vi "Digital Telemetry.vi"() -> ()   [LabVIEW 2020]
uses:
  <vilib>/MakerHub/LINX/Private/Type Defs/Peripheral.ctl
  <vilib>/MakerHub/LINX/Public/Peripherals/Digital/Digital Read 1 Chan.vi
  <vilib>/MakerHub/LINX/Public/Peripherals/Digital/Digital Write 1 Chan.vi
  <vilib>/MakerHub/LINX/Public/Peripherals/Digital/Digital Read N Chans.vi
  <vilib>/MakerHub/LINX/Public/Peripherals/Digital/Digital Write N Chans.vi
  <vilib>/MakerHub/LINX/Private/Local IO/LinxDigitalRead.vi
  <vilib>/MakerHub/LINX/Private/Local IO/LinxDigitalWrite.vi
  <vilib>/MakerHub/LINX/Public/Utilities/Open Local.vi
  <vilib>/MakerHub/LINX/Private/Utilties/Generate Error.vi
  <vilib>/MakerHub/LINX/LMH-LINX.lvlib
panel:
  out "Error Out 3":errorcluster
  out "Numeric":i32
  in  "DO Channel":u8
  out "Error Out":errorcluster
  in  "Write Value?":bool
  in  "Write All?":bool
  in  "Output Value":bool
  out "Numeric 2":u8
  out "Error Out 2":errorcluster
  out "Values":bool[](array[boolean])
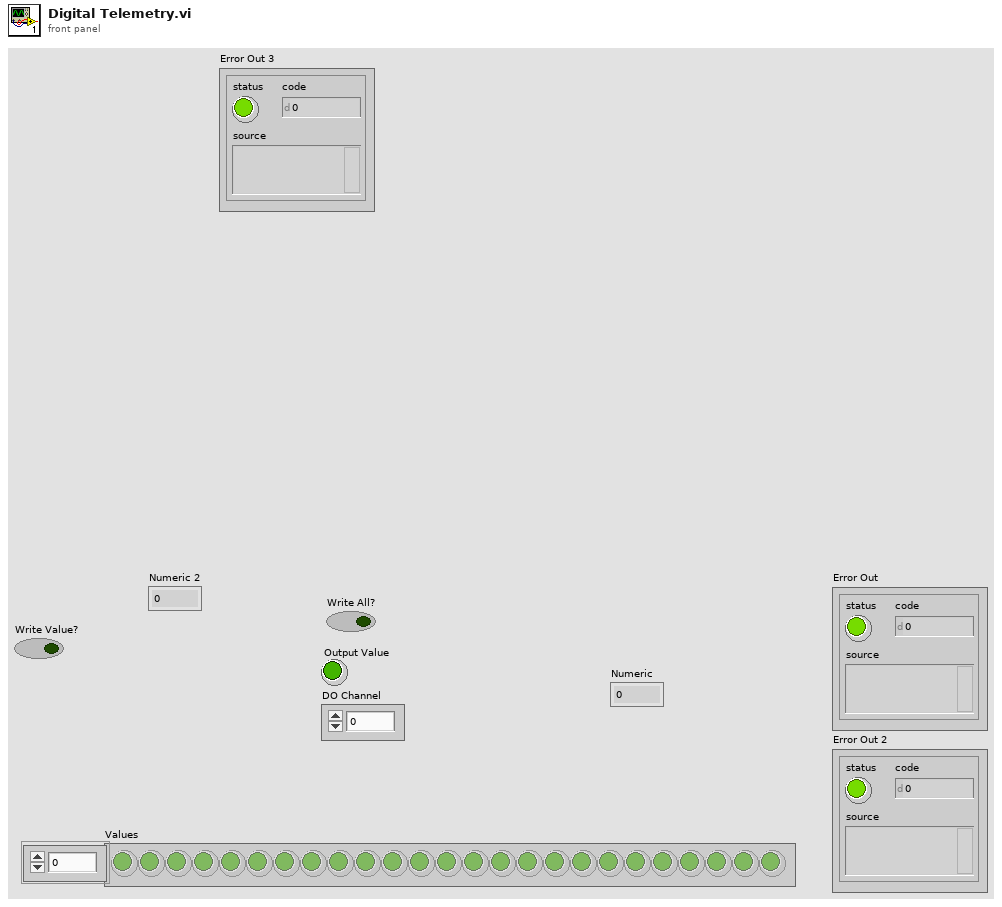
[diagram p1: front panel]
types:
  T1 = typedef "LMH-LINX.lvlib/LINX Ref.ctl" = cluster{"IO":T2, "Interface":T3, "LINX Device Config":T4}
  T2 = typedef "LMH-LINX.lvlib/Platform.ctl" = enum16{"Remote", "Local"}
  T3 = typedef "LMH-LINX.lvlib/Interface.ctl" = enum16{"Serial", "TCP"}
  T4 = typedef "LMH-LINX.lvlib/Device.lvlib/LINX Device Config.ctl" = cluster{"Interface":T3, "COM Port":refnum<visa-resource-name>, "TCP Configuration":T5, "Device Family":u8, "Device ID":u8, "Device Name":string, "TCP Ref":refnum<k5>, "Channels":T6}
  T5 = typedef "LMH-LINX.lvlib/Device.lvlib/TCP Config.ctl" = cluster{"IP Address":string, "Port":u16}
  T6 = typedef "LMH-LINX.lvlib/Channels.ctl" = cluster{"DI":u8[], "DO":u8[], "AI":u8[], "AO":u8[], "PWM":u8[], "QE":u8[], "UART":u8[], "I2C 2":u8[], "SPI":u8[], "CAN":u8[], "Servo":u8[], "AI Ref (V)":dbl, "AI Resolution (Bits)":u8, "AO Ref (V)":dbl, "AO Resolution (Bits)":u8}
  T7 = typedef "LMH-LINX.lvlib/Peripheral.ctl" = enum8{"DI", "DO", "AI", "AO", "PWM", "QE", "UART", "I2C", "SPI", "CAN", "Servo"}
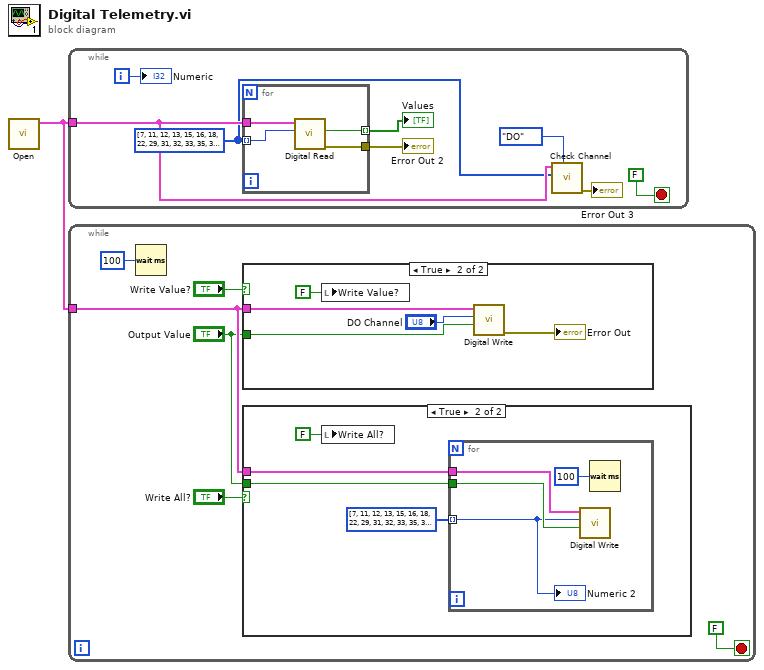
[diagram p0: block diagram]
diagram:
  n1 = call-poly <vilib>:"Open.vi"() -> ("LINX Resource"=w1:T1)  [unwired: 9 in, 2 out]
  n2 = while {
    tunnel: w1 -> [w4]
    i -> [w6]
    stop <- FALSE stop-if-true
    w2 = u8[] [7, 11, 12, 13, 15, 16, 18, 22, 29, 31, 32, 33, 35, 36, 37, 38, 40] ("DI Channels")
    n3 = for {
      tunnel: [w13] -> w9 mode=indexing
      tunnel: [w12] -> w8
      tunnel: w2 -> [w11] mode=indexing
      tunnel: w4 -> [w10]
      n4 = call-poly <vilib>:"Digital Read.vi"("DI Channel"=w11, "LINX Resource"=w10) -> ("Error Out"=w12:errorcluster, "DI Value"=w13:bool)  [unwired: 7 in, 1 out]
    }
    "Values" <- w9
    "Error Out 2" <- w8
    n5 = call <vilib>:"Check Channel.vi"("Peripheral"=Peripheral."DO", "Channels"=w2, "LINX Resource"=w4) -> ("Error Out"=→"Error Out 3":errorcluster)  [unwired: 6 in, 2 out]
    "Numeric" <- w6
  }
  n6 = while {
    tunnel: w1 -> [w16]
    stop <- FALSE stop-if-true
    n7 = Wait (ms)(milliseconds to wait=u32 100) -> ()  [unwired: 1 out]
    n8 = case shown="True" "Write Value?" {
      tunnel: w16 -> [_ w32]
      tunnel: "Output Value" -> [_ w28]
      frame False {
      }
      frame True {
        n9 = local write "Write Value?"(FALSE ("Write Value?")) -> ()
        n10 = call-poly <vilib>:"Digital Write.vi"("Output Value"=w28, "DO Channel"="DO Channel", "LINX Resource"=w32) -> ("Error Out"=→"Error Out":errorcluster)  [unwired: 7 in, 1 out]
      }
    }
    n11 = case shown="True" "Write All?" {
      tunnel: w16 -> [_ w23]
      tunnel: "Output Value" -> [_ w22]
      frame False {
      }
      frame True {
        n12 = local write "Write All?"(FALSE ("Write Value?")) -> ()
        n13 = for {
          tunnel: w23 -> [w27]
          tunnel: w22 -> [w26]
          tunnel: u8[] [7, 11, 12, 13, 15, 16, 18, 22, 29, 31, 32, 33, 35, 36, 37, 38, 40] ("DI Channels") -> [w24] mode=indexing
          n14 = call-poly <vilib>:"Digital Write.vi"("Output Value"=w26, "DO Channel"=w24, "LINX Resource"=w27) -> ()  [unwired: 7 in, 2 out]
          n15 = Wait (ms)(milliseconds to wait=u32 100) -> ()  [unwired: 1 out]
          "Numeric 2" <- w24
        }
      }
    }
  }
